vi "0037-0002_HDC1080.vi"() -> ()   [LabVIEW 2014]
panel:
  out "相対湿度":dbl format="%#.3g"
  out "温度":dbl format="%#.3g"
  out "error out":errorcluster caption="エラー出力"
  in  "停止ボタン":bool
  # "℃"
  # "％RH"
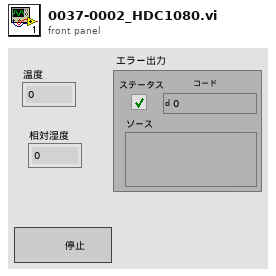
[diagram p1: front panel]
types:
  T1 = cluster{"bitRate":u32, "address":u8, "autoReadRespond":bool, "writeTimeout":u16, "readTimeout":u16, "sclLowTimeout":bool, "transferRetries":u16}
  T2 = typedef "CP2112_device.ctl" = i32
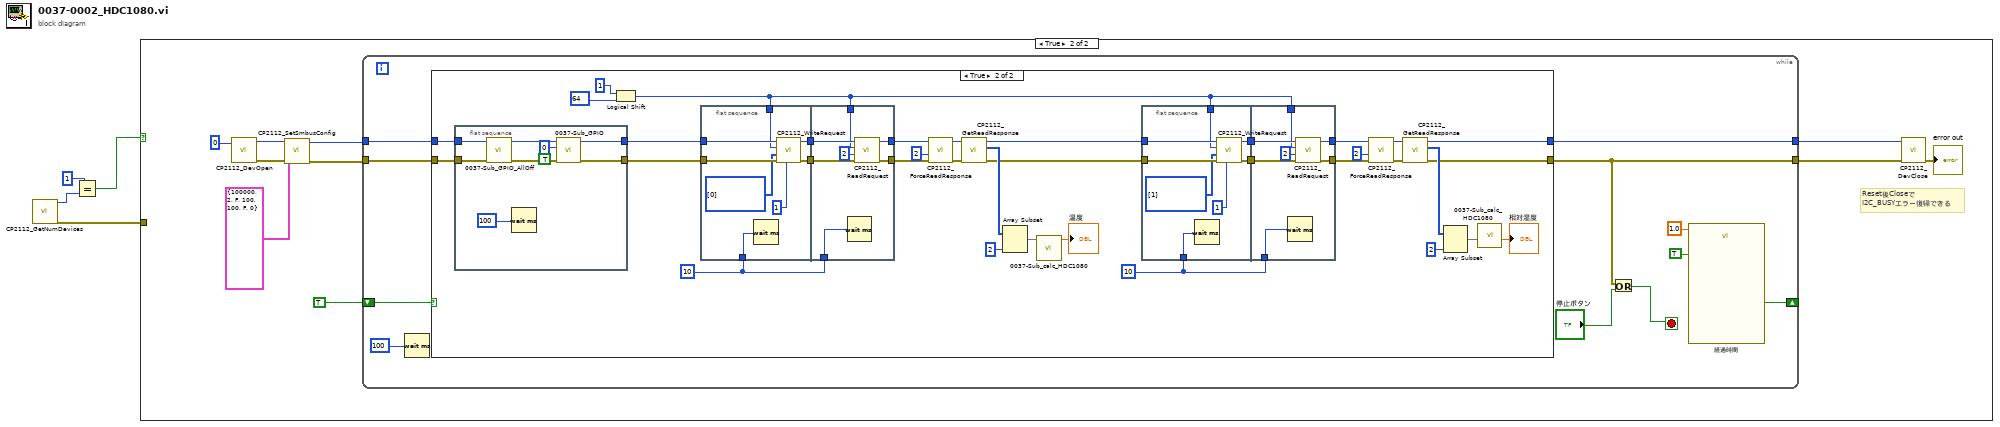
[diagram p0: block diagram]
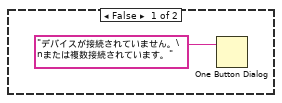
[diagram p2: hidden frame]
diagram:
  n1 = call "CP2112_GetNumDevices.vi"() -> ("error out"=w1:errorcluster, "numDevices"=w3:i32)  [unwired: 9 in, 1 out]
  n2 = Equal?(x=1, y=w3) -> (x = y?=w2:bool)
  n3 = case shown="TRUE" w2 {
    tunnel: w1 -> [_ _]
    frame False {
      n4 = One Button Dialog(message="デバイスが接続されていません。\nまたは複数接続されています。" ("メッセージ")) -> ()  [unwired: 1 in, 1 out]
    }
    frame True {
      # "Reset後Closeで\nI2C_BUSYエラー復帰できる"
      n5 = call "CP2112_DevOpen.vi"("deviceNum"=0) -> ("error out"=w10:errorcluster, "device"=w11:T2)  [unwired: 8 in, 1 out]
      n6 = call "CP2112_SetSmbusConfig.vi"("error in (no error)"=w10, "smbusInfo"=T1 {"bitRate"=100000, "address"=2, "autoReadRespond"=FALSE, "writeTimeout"=100, "readTimeout"=100, "sclLowTimeout"=FALSE, "transferRetries"=0}, "device"=w11) -> ("error out"=w12:errorcluster, "deviceOut"=w13:T2)  [unwired: 6 in, 1 out]
      n7 = while {
        tunnel: w12 -> [w26]
        tunnel: w13 -> [w25]
        tunnel: [w22] -> w8
        tunnel: [w21] -> w7
        shift-right: [w18] -> _
        shift-left: TRUE ("Auto Reset") -> [w19]
        stop <- w23 stop-if-true
        n8 = Wait (ms)(milliseconds to wait=u32 100 ("ミリ秒待機時間")) -> ()  [unwired: 1 out]
        n9 = case shown="TRUE" w19 {
          tunnel: w26 -> [w27 w52]
          tunnel: w25 -> [w28 w53]
          tunnel: [w27 w34] -> w22
          tunnel: [w28 w35] -> w21
          frame False {
          }
          frame True {
            w38 = u32 10 ("ミリ秒待機時間")
            w54 = u32 10 ("ミリ秒待機時間")
            n10 = flat-sequence {
              tunnel: w53 -> [w87]
              tunnel: w52 -> [w84]
              tunnel: [w85] -> w48
              tunnel: [w82] -> w49
              frame #0 {
                n11 = call "0037-Sub_GPIO_AllOff.vi"("エラー出力 2"=w84, "device"=w87) -> ("エラー出力"=w83:errorcluster, "deviceOut"=w86:T2)  [unwired: 8 in]
                n12 = Wait (ms)(milliseconds to wait=u32 100 ("ミリ秒待機時間")) -> ()  [unwired: 1 out]
                n13 = call "0037-Sub_GPIO.vi"("エラー出力 2"=w83, "ブール"=TRUE, "GPIO"=u8 0, "device"=w86) -> ("エラー出力"=w82:errorcluster, "deviceOut"=w85:T2)  [unwired: 6 in]
              }
            }
            n14 = Logical Shift(y=1, x=64) -> (x << y=w33:i32)
            n15 = flat-sequence {
              tunnel: w49 -> [w95]
              tunnel: w48 -> [w94]
              tunnel: w33 -> [w89]
              tunnel: [w93] -> w58
              tunnel: [w92] -> w57
              tunnel: w54 -> [w88]
              tunnel: w58 -> [w100]
              tunnel: w57 -> [w99]
              tunnel: [w101] -> w56
              tunnel: [w98] -> w55
              tunnel: w33 -> [w97]
              tunnel: w54 -> [w96]
              frame #0 {
                n16 = Wait (ms)(milliseconds to wait=w88) -> ()  [unwired: 1 out]
                n17 = call "CP2112_WriteRequest.vi"("numBytesToWrite"=i16 1 ("numByteToRead"), "error in (no error)"=w95, "buffer"=u8[] [0], "slaveAddress"=w89, "device"=w94) -> ("error out"=w93:errorcluster, "deviceOut"=w92:T2)  [unwired: 4 in, 1 out]
              }
              frame #1 {
                n18 = Wait (ms)(milliseconds to wait=w96) -> ()  [unwired: 1 out]
                n19 = call "CP2112_ReadRequest.vi"("error in (no error)"=w100, "numByteToRead"=i16 2, "slaveAddress"=w97, "device"=w99) -> ("error out"=w101:errorcluster, "deviceOut"=w98:T2)  [unwired: 5 in, 1 out]
              }
            }
            n20 = call "CP2112_ForceReadResponse.vi"("error in (no error)"=w56, "numByteToRead"=i16 2, "device"=w55) -> ("error out"=w63:errorcluster, "deviceOut"=w62:T2)  [unwired: 6 in, 1 out]
            n21 = call "CP2112_GetReadResponse.vi"("error in (no error)"=w63, "device"=w62) -> ("error out"=w36:errorcluster, "buffer"=w60:u8[], "deviceOut"=w37:T2)  [unwired: 4 in, 3 out]
            n22 = Array Subset(array=w60, length=2 ("長さ")) -> (w32:u8[])  [unwired: 1 in]
            n23 = call "0037-Sub_calc_HDC1080.vi"("temp"=w32) -> ("temp"=→"温度":dbl)  [unwired: 8 in, 1 out]
            n24 = flat-sequence {
              tunnel: w36 -> [w71]
              tunnel: w37 -> [w70]
              tunnel: w33 -> [w65]
              tunnel: [w69] -> w47
              tunnel: [w68] -> w46
              tunnel: w38 -> [w64]
              tunnel: w47 -> [w76]
              tunnel: w46 -> [w75]
              tunnel: [w77] -> w40
              tunnel: [w74] -> w39
              tunnel: w33 -> [w73]
              tunnel: w38 -> [w72]
              frame #0 {
                n25 = Wait (ms)(milliseconds to wait=w64) -> ()  [unwired: 1 out]
                n26 = call "CP2112_WriteRequest.vi"("numBytesToWrite"=i16 1 ("numByteToRead"), "error in (no error)"=w71, "buffer"=u8[] [1], "slaveAddress"=w65, "device"=w70) -> ("error out"=w69:errorcluster, "deviceOut"=w68:T2)  [unwired: 4 in, 1 out]
              }
              frame #1 {
                n27 = Wait (ms)(milliseconds to wait=w72) -> ()  [unwired: 1 out]
                n28 = call "CP2112_ReadRequest.vi"("error in (no error)"=w76, "numByteToRead"=i16 2, "slaveAddress"=w73, "device"=w75) -> ("error out"=w77:errorcluster, "deviceOut"=w74:T2)  [unwired: 5 in, 1 out]
              }
            }
            n29 = call "CP2112_ForceReadResponse.vi"("error in (no error)"=w40, "numByteToRead"=i16 2, "device"=w39) -> ("error out"=w45:errorcluster, "deviceOut"=w44:T2)  [unwired: 6 in, 1 out]
            n30 = call "CP2112_GetReadResponse.vi"("error in (no error)"=w45, "device"=w44) -> ("error out"=w34:errorcluster, "buffer"=w42:u8[], "deviceOut"=w35:T2)  [unwired: 4 in, 3 out]
            n31 = Array Subset(array=w42, length=2 ("長さ")) -> (w30:u8[])  [unwired: 1 in]
            n32 = call "0037-Sub_calc_HDC1080.vi"("humi"=w30) -> ("humi"=→"相対湿度":dbl)  [unwired: 8 in, 1 out]
          }
        }
        n33 = Or(x=w22, y="停止ボタン") -> (x .or. y?=w23:bool)
        n34 = call "経過時間"("Time Target (s)"=1.0, "Auto Reset"=TRUE) -> ("Time has Elapsed"=w18:bool)  [unwired: 10 in, 7 out]
      }
      n35 = call "CP2112_DevClose.vi"("error in (no error)"=w8, "device"=w7) -> ("error out"=→"error out":errorcluster)  [unwired: 9 in]
    }
  }
